vi "Insert Element at End.vi"(8 "error in (no error)":errorcluster, 9 "element":variant, 10 "Name":string, 11 "Cluster in":variant) -> (0 "error out":errorcluster, 3 "Cluster out":variant)   [LabVIEW 2017, in "Variant Data Manipulation.lvlib"]
uses:
  Variant Data Manipulation.lvlib
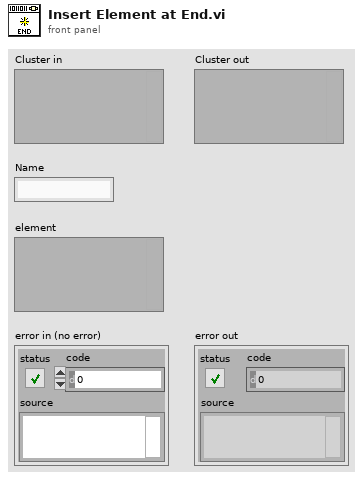
[diagram p1: front panel]
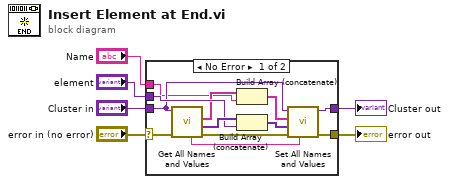
[diagram p0: block diagram]
diagram:
  n1 = case shown="No Error" "error in (no error)" {
    selector: "error in (no error)" -> [w18 w19]
    tunnel: [w15 w19] -> w5
    tunnel: [w14 w20] -> w4
    tunnel: "element" -> [w12 _]
    tunnel: "Cluster in" -> [w11 w20]
    tunnel: "Name" -> [w9 _]
    frame No Error {
      n2 = call "Get All Names and Values.vi"("error in"=w18, "Cluster in"=w11) -> ("error out"=w16:errorcluster, "Values"=w17:variant[], "Element Names"=w10:string[], "Cluster Name"=w7:string)  [unwired: 5 in, 1 out]
      n3 = Build Array (concatenate)(w10, w9) -> (w8:string[])
      n4 = Build Array (concatenate)(w17, w12) -> (w13:variant[])
      n5 = call "Set All Names and Values.vi"("Cluster Name"=w7, "error in"=w16, "values"=w13, "Element Names"=w8, "Cluster in"=w11) -> ("error out"=w15:errorcluster, "Cluster out"=w14:variant)  [unwired: 5 in]
    }
    frame Error {
    }
  }
  "Cluster out" <- w4
  "error out" <- w5
